vi "save_counter_data.vi"(7 "Counter Settings, Tasks and Data":T1, 8 "error in (no error)":errorcluster, 9 "counter data":u32[][][](array[numeric]), 10 "XYZC iteration string":string, 11 "Data Files Path":path=path "C:/Users/QCC/Documents/Cesium_project/LabVIEW Projects/data/2011_03_02") -> (0 "error out":errorcluster)   [LabVIEW 2013]
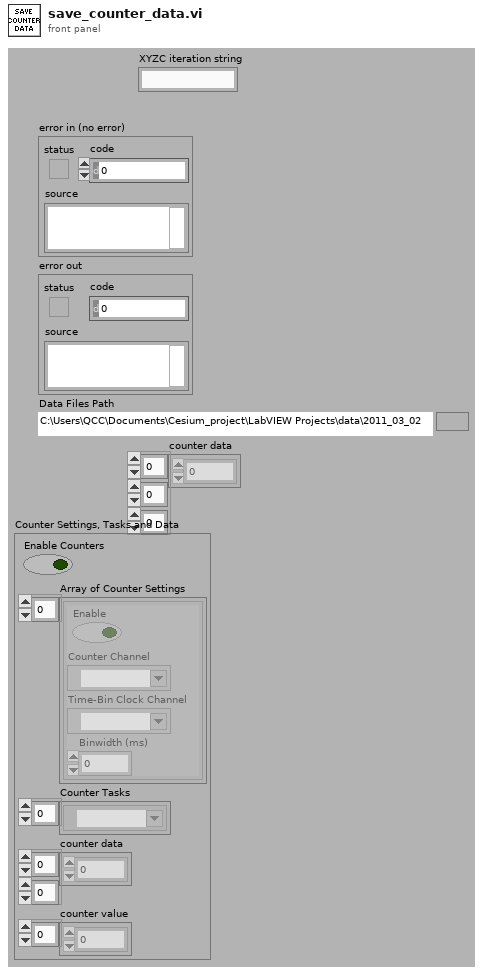
[diagram p1: front panel]
types:
  T1 = cluster{"Enable Counters":bool, "Array of Counter Settings":cluster{"Enable":bool, "Counter Channel":tag, "Time-Bin Clock Channel":tag, "Binwidth (ms)":dbl}[], "Counter Tasks":refnum<k21>[], "counter data":u32[][], "counter value":u32[]}
  T2 = cluster{"Enable":bool, "Counter Channel":tag, "Time-Bin Clock Channel":tag, "Binwidth (ms)":dbl}[]
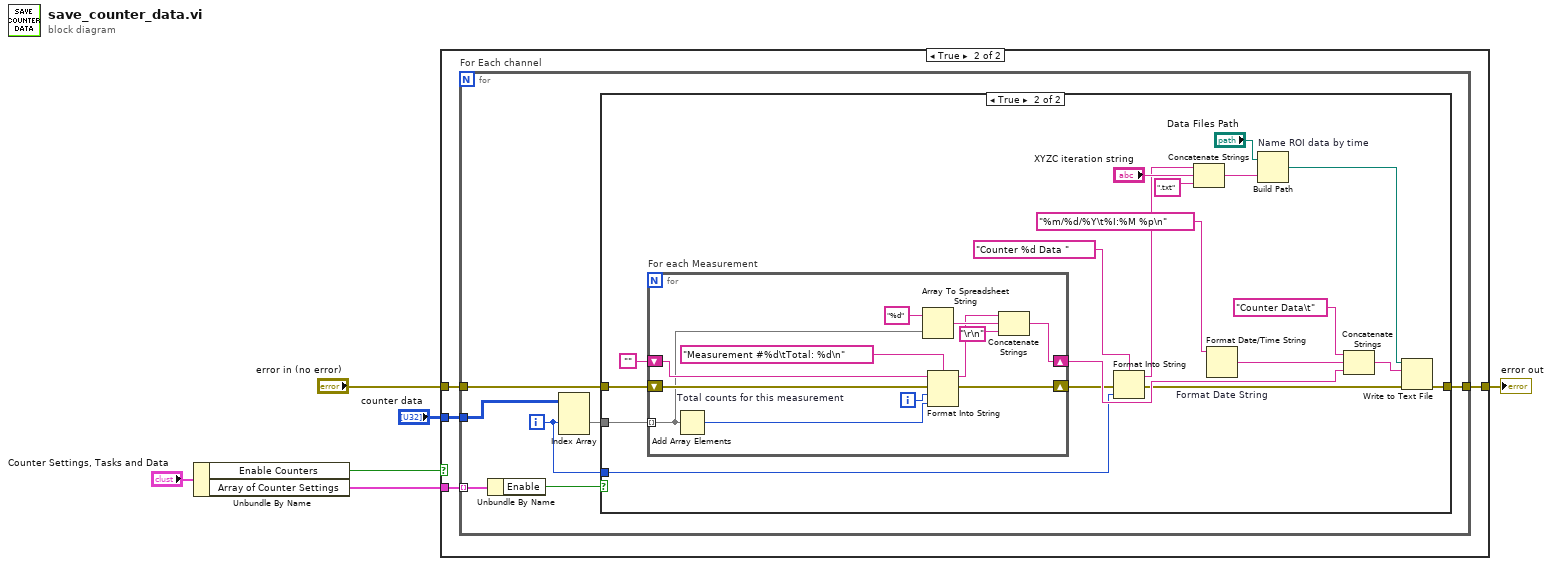
[diagram p0: block diagram]
diagram:
  n1 = Unbundle By Name("Counter Settings, Tasks and Data") -> ("Enable Counters"=w2:bool, "Array of Counter Settings"=w1:T2)
  n2 = case shown="True" w2 {
    tunnel: "counter data" -> [_ w8]
    tunnel: "error in (no error)" -> [w7 w11]
    tunnel: [w7 w10] -> w4
    tunnel: w1 -> [_ w9]
    frame False {
    }
    frame True {
      n3 = for "For Each channel" {
        tunnel: w11 -> [w18]
        tunnel: [w17] -> w10
        tunnel: w9 -> [w16] mode=indexing
        tunnel: w8 -> [w14]
        i -> [w12]
        n4 = Unbundle By Name(w16) -> ("Enable"=w15:bool)
        n5 = Index Array(array=w14, index (dim 1)=w12) -> (element=w13:u32[][])  [unwired: 2 in]
        n6 = case shown="True" w15 {
          tunnel: w13 -> [_ w27]
          tunnel: w12 -> [_ w25]
          tunnel: w18 -> [w19 w24]
          tunnel: [w19 w23] -> w17
          frame False {
          }
          frame True {
            n7 = for "For each Measurement" {
              shift-right: [w47] -> w21
              shift-left: w24 -> [w48]
              shift-right: [w41] -> w32
              shift-left: "" -> [w46]
              tunnel: w27 -> [w40] mode=indexing
              i -> [w49]
              n8 = Add Array Elements "Total counts for this measurement"(numeric array=w40) -> (sum=w39:u32)
              n9 = Array To Spreadsheet String(array=w40, 3:"%d" ("format string")) -> (spreadsheet string=w44:string)  [unwired: 1 in]
              n10 = Format Into String(format string="Measurement #%d\tTotal: %d\n", initial string=w46, error in=w48, w49, w39) -> (resulting string=w43:string, error out=w47:errorcluster)
              n11 = Concatenate Strings(w43, w44, "\r\n") -> (w41:string)
            }
            n12 = Format Into String(format string="Counter %d Data ", error in=w21, w25) -> (resulting string=w22:string, error out=w20:errorcluster)  [unwired: 1 in]
            n13 = Concatenate Strings(w22, "XYZC iteration string", ".txt" ("string")) -> (w37:string)
            n14 = Format Date/Time String "Format Date String"(time format string (%c)="%m/%d/%Y\t%I:%M %p\n") -> (date/time string=w30:string)  [unwired: 2 in]
            n15 = Build Path "Name ROI data by time"(base path="Data Files Path", name or relative path=w37) -> (appended path=w38:path)
            n16 = Concatenate Strings("Counter Data\t", w30, w32) -> (w29:string)
            n17 = Write to Text File(file (use dialog)=w38, text=w29, error in=w20) -> (error out=w23:errorcluster)  [unwired: 1 in, 2 out]
          }
        }
      }
    }
  }
  "error out" <- w4
